vi "EX 6-4  Thumb Stick RGB LED.vi"() -> ()   [LabVIEW 2011, in "LabVIEW Interface for Arduino.lvlib"]
doc: "An example that uses an Arduino to capture input from an analog thumb stick which is used to generate colors based on the angle and magnitude of the thumb stick. These colors are displayed on the front panel and sent to an RGB LED . (The RGB LED can easily be replaced with BlinkMs)"
uses:
  <vilib>/LabVIEW Interface for Arduino/LabVIEW Interface for Arduino.lvlib
panel:
  out "Color":u32(colorbox)=1297
  out "Vertical Axis":dbl(slide)=2.3226 scale=0.0..5.0
  out "Horizontal Axis":dbl(slide)=2.3863 scale=0.0..5.0
  in  "Stop":bool
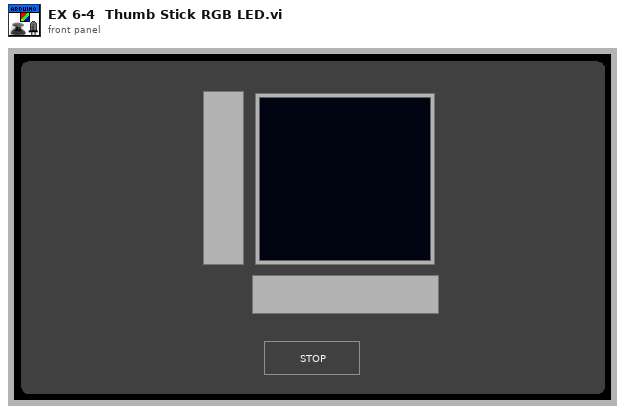
[diagram p1: front panel]
types:
  T1 = typedef "LabVIEW Interface for Arduino.lvlib/Arduino Resource.ctl" = cluster{"VISA resource":refnum<visa-resource-name>, "Board Type":T2, "Connection Type":enum8{"USB / Serial"}, "Bytes Per Packet (15)":u8}
  T2 = typedef "LabVIEW Interface for Arduino.lvlib/Board Type.ctl" = enum16{"Uno", "Dimuelanove w/Atmega 328", "Mega 2560"}
  T3 = cluster{"Horizontal Axis Pin":dbl, "Vertical Axis Pin":dbl, "Select Pin":dbl}
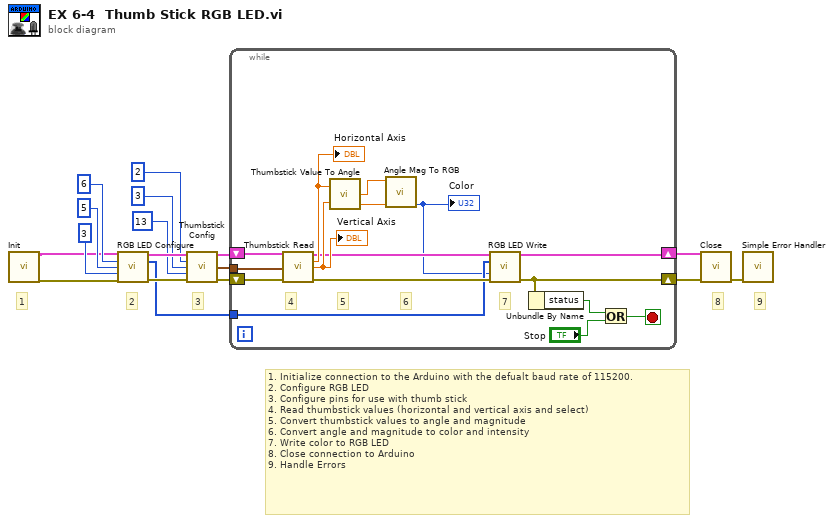
[diagram p0: block diagram]
diagram:
  # "9"
  # "8"
  # "3"
  # "2"
  # "1"
  # "1. Initialize connection to the Arduino with the defualt baud rate of 115200.\n2. Configure RGB LED\n3. Configure pins for use with thumb stick\n4. Read thumbstick values (horizontal and vertical axis and select)\n5. Convert thumbstick values to angle and magnitude\n6. Convert angle and magnitude to color and intensity\n7. Write color to RGB LED\n8. Close connection to Arduino\n9. Handle Errors"
  n1 = call <vilib>:"Init.vi"() -> ("Arduino Resource"=w2:T1, "error out"=w1:errorcluster)  [unwired: 18 in]
  n2 = call <vilib>:"RGB LED Configure.vi"("Arduino Resource"=w2, "Red Pin"=u8 6, "Green Pin"=u8 5, "Blue Pin"=u8 3, "error in"=w1) -> ("Arduino Resource"=w12:T1, "RGB LED Pins"=w3:u8[], "error out"=w11:errorcluster)  [unwired: 8 in]
  n3 = call <vilib>:"Thumbstick Config.vi"("Arduino Resource"=w12, "Horizontal Axis AI Pin"=u8 2, "Vertical Axis AI Pin"=u8 3, "Select DI Pin"=u8 13, "error in"=w11) -> ("Arduino Resource"=w16:T1, "Thumbstick Data"=w17:T3, "error out"=w15:errorcluster)  [unwired: 8 in]
  n4 = while {
    shift-right: [w19] -> w5
    shift-left: w16 -> [w33]
    shift-right: [w18] -> w14
    shift-left: w15 -> [w32]
    tunnel: w17 -> [w31]
    tunnel: w3 -> [w21]
    stop <- w23 stop-if-true
    # "7"
    # "6"
    # "5"
    # "4"
    n5 = call <vilib>:"Thumbstick Read.vi"("Arduino Resource"=w33, "Thumbstick Data"=w31, "error in"=w32) -> ("Arduino Resource"=w22:T1, "Horizontal Axis"=w28:dbl, "Vertical Axis"=w27:dbl, "error out"=w26:errorcluster)  [unwired: 8 in, 1 out]
    "Horizontal Axis" <- w28
    "Vertical Axis" <- w27
    n6 = call <vilib>:"Thumbstick Value To Angle.vi"("Vertical Axis"=w27, "Horizontal Axis"=w28) -> ("Magnitude"=w30:dbl, "Degrees"=w29:dbl)  [unwired: 1 out]
    n7 = call <vilib>:"Angle Mag To RGB.vi"("Magnitude (0-1)"=w30, "Angle (Degrees)"=w29) -> ("RGB Color"=w20:u32)  [unwired: 6 in, 3 out]
    "Color" <- w20
    n8 = call <vilib>:"RGB LED Write.vi"("Arduino Resource"=w22, "RGB LED Pins"=w21, "Color"=w20, "error in"=w26) -> ("Arduino Resource"=w19:T1, "error out"=w18:errorcluster)  [unwired: 9 in, 1 out]
    n9 = Unbundle By Name(w18) -> ("status"=w25:bool)
    n10 = Or(x=w25, y="Stop") -> (x .or. y?=w23:bool)
  }
  n11 = call <vilib>:"Close.vi"("Arduino Resource"=w5, "error in"=w14) -> ("error out"=w13:errorcluster)  [unwired: 13 in]
  n12 = call <vilib>:"Simple Error Handler.vi"("error in (no error)"=w13) -> ()  [unwired: 4 in, 5 out]
